vi "Graph Tool Testing1.vi"() -> ()   [LabVIEW 2019]
uses:
  Support/Graph Tools/Selection VIs/controls/CursorOptions.ctl
  <vilib>/Utility/miscctls.llb/LVRectTypeDef.ctl
  Support/Graph Tools/Selection VIs/controls/MarkerInfo.ctl
  Support/Graph Tools/Selection VIs/controls/markerType.ctl
  Support/Graph Tools/[Selection] Config.ctl
  <vilib>/Utility/miscctls.llb/LVPoint32TypeDef.ctl
  Support/Graph Tools/[Comment] Actions.ctl
  Support/Graph Tools/Selection Y-axis.vi
  Support/Graph Tools/Selection X-axis.vi
  Support/Graph Tools/Graph Tools.lvlib
panel:
  out "Display:Primary Workspace":T1
  out "Output Valid":bool
  out "X2":dbl
  out "X1":dbl
  in  "picture":picture
  in  "Cursor Options":T2={"font"={"Font Name"="Arial", "Size"=14, "Strikeout?"=FALSE, "Italic?"=FALSE, "Underline?"=FALSE, "Outline?"=FALSE, "Shadow?"=FALSE, "Bold?"=FALSE}, "size"=1, "Timestamp"=enum."at TOP", "Vertical Line?"=FALSE, "Horizontal Line?"=FALSE, "alignment(left, top)"={"horizontal"=enum."center", "vertical"=enum."center"}, "TextFormat"="%.3p %.3p %s", "time format (%H:%M:%S)"="%H:%M%:S"} {"size" min=1 max=50}
  out "Waveform Graph":T3(graph)
  out "XY Graph":cluster{i32[], dbl[]}[](graph)
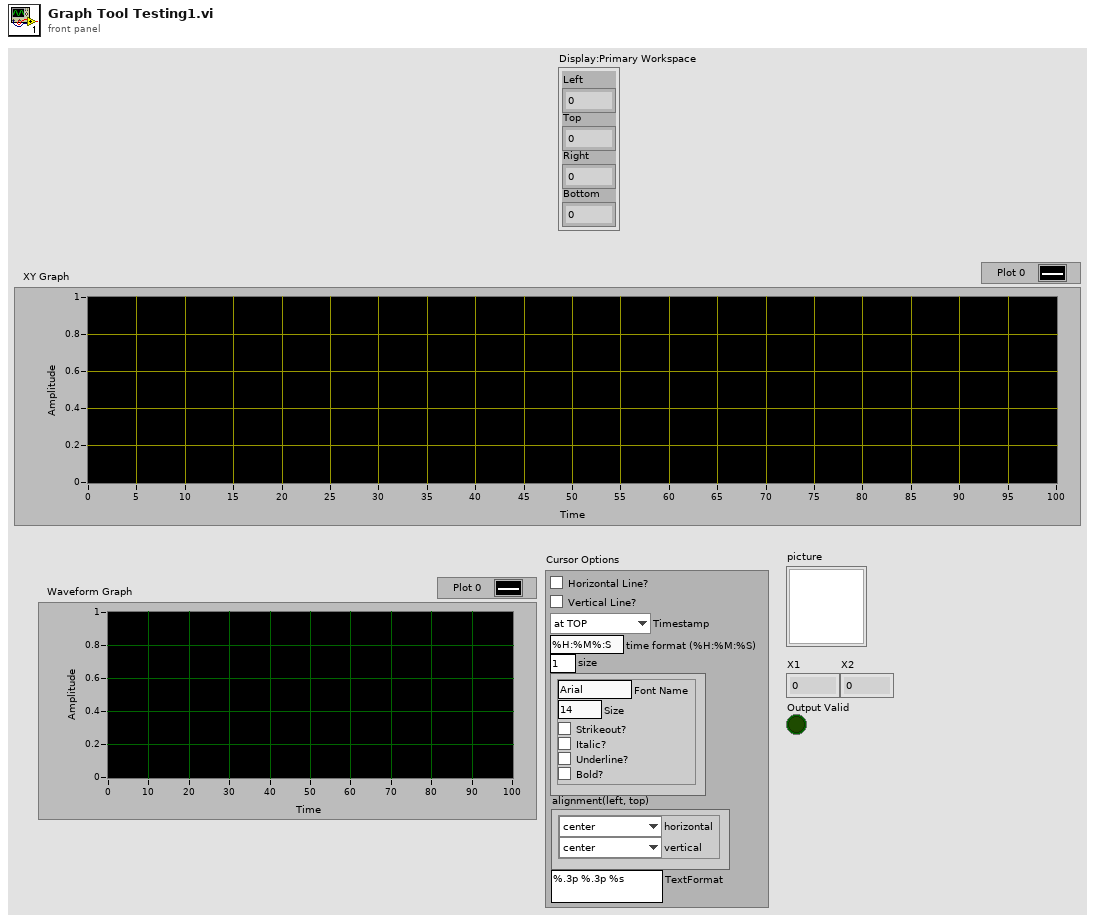
[diagram p1: front panel]
types:
  T1 = typedef "LVRectTypeDef.ctl" = cluster{"Left":i16, "Top":i16, "Right":i16, "Bottom":i16}
  T2 = typedef "CursorOptions.ctl" = cluster{"font":cluster{"Font Name":string, "Size":i16, "Strikeout?":bool, "Italic?":bool, "Underline?":bool, "Outline?":bool, "Shadow?":bool, "Bold?":bool}, "size":i16, "Timestamp":enum16{"at TOP", "at BOTTOM", "none"}, "Vertical Line?":bool, "Horizontal Line?":bool, "alignment(left, top)":cluster{"horizontal":enum16{"left", "center", "right"}, "vertical":enum16{"top", "center", "bottom"}}, "TextFormat":string, "time format (%H:%M:%S)":string}
  T3 = cluster{"number (0 to 1)":dbl, "number (0 to 1)":dbl, dbl[]}[]
  T4 = typedef "MarkerInfo.ctl" = cluster{"Type":T5, "X":dbl, "Y":dbl, "X2":dbl, "Y2":dbl, "Text":string}
  T5 = typedef "markerType.ctl" = enum16{"point", "arrow", "horiz", "vert", "vert range", "horiz range", "box"}
  T6 = cluster{"number (0 to 1)":dbl, "number (0 to 1)":dbl, dbl[]}
  T7 = typedef "Graph Tools.lvlib/[Comment] Actions.ctl" = enum16{"New Comment", "Refresh", "Clear", "Stop", "Test"}
  T8 = typedef "Graph Tools.lvlib/[Selection] Config.ctl" = cluster{"Selection":cluster{"caption":string, "Validaty Threshold":i32, "Color":u32, "Start Coords":T9}}
  T9 = typedef "LVPoint32TypeDef.ctl" = cluster{"Horizental":i32, "Vertical":i32}
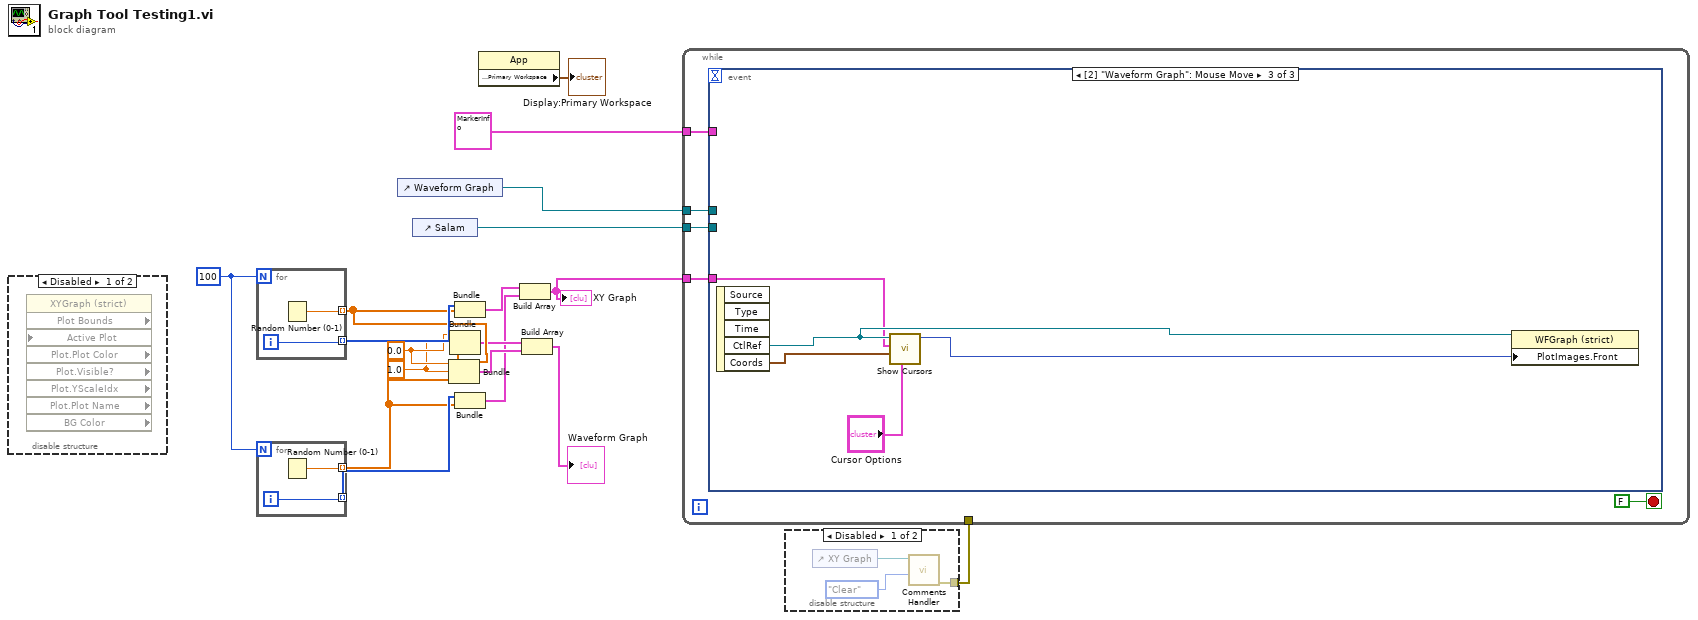
[diagram p0: block diagram]
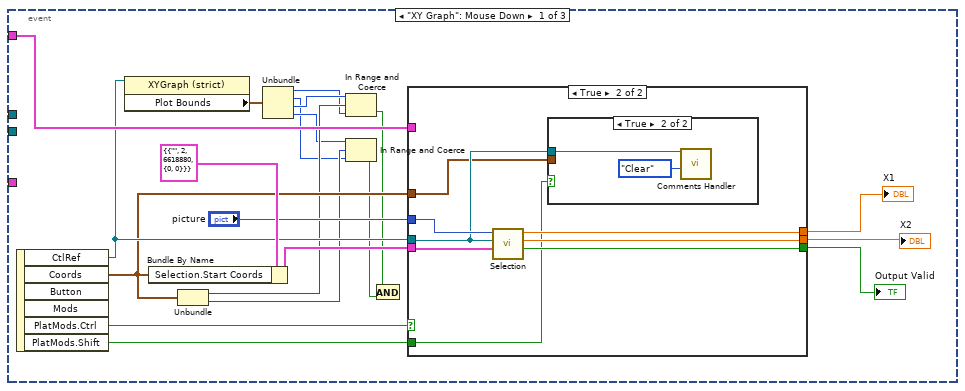
[diagram p4: hidden frame]
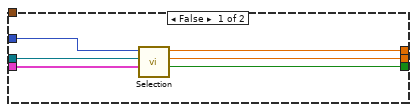
[diagram p5: hidden frame]
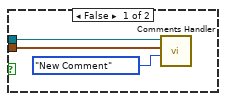
[diagram p6: hidden frame]
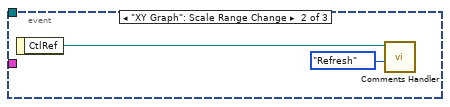
[diagram p7: hidden frame]
diagram:
  w10 = 1.0 ("number (0 to 1)")
  w11 = 0.0 ("number (0 to 1)")
  w16 = 100
  n1 = disable-structure shown="Disabled" {
    frame Disabled {
      n2 = property on="Property Node" class="XYGraph (strict)" props=["Plot Bounds", "Active Plot", "Plot", "Plot Color", "Plot", "Visible?", "Plot", "YScaleIdx", "Plot", "Plot Name", "BG Color"]() -> ()  [unwired: 3 in, 8 out]
    }
    frame Enabled {
    }
  }
  n3 = for {
    N: w16 -> [_]
    tunnel: [w20] -> w18 mode=indexing
    tunnel: [w19] -> w9 mode=indexing
    i -> [w20]
    n4 = Random Number (0-1)() -> (number: 0 to 1=w19:dbl)
  }
  n5 = for {
    N: w16 -> [_]
    tunnel: [w22] -> w17 mode=indexing
    tunnel: [w21] -> w13 mode=indexing
    i -> [w22]
    n6 = Random Number (0-1)() -> (number: 0 to 1=w21:dbl)
  }
  n7 = control-ref of="Waveform Graph"() -> (w6:refnum<vi>)
  n8 = control-ref of="Salam"() -> (w14:refnum<vi>)
  n9 = Bundle("number (0 to 1)"=w11, "number (0 to 1)"=w10, w13) -> (w12:T6)  [unwired: 1 in]
  n10 = Bundle("number (0 to 1)"=w11, "number (0 to 1)"=w10, w9) -> (w8:T6)  [unwired: 1 in]
  n11 = Bundle(w18, w9) -> (w15:cluster{i32[], dbl[]})  [unwired: 1 in]
  n12 = Bundle(w17, w13) -> (w7:cluster{i32[], dbl[]})  [unwired: 1 in]
  n13 = property class="App"() -> ("Display:Primary Workspace"=→"Display:Primary Workspace":T1)  [unwired: 2 in, 2 out]
  n14 = Build Array(w15, w7) -> (w4:cluster{i32[], dbl[]}[])
  "XY Graph" <- w4
  n15 = Build Array(w8, w12) -> (→"Waveform Graph":T3)
  n16 = disable-structure shown="Disabled" {
    disable-tunnel: [w23 _] -> w1
    frame Disabled {
      n17 = control-ref of="XY Graph"() -> (w25:refnum<vi>)
      n18 = call "Comments Handler.vi"("Action"=[Comment]_Actions."Clear", "GrphChrt"=w25) -> ("error out"=w23:errorcluster)  [unwired: 9 in]
    }
    frame Enabled {
    }
  }
  n19 = while {
    tunnel: w14 -> [w29]
    tunnel: w6 -> [w28]
    tunnel: w4 -> [w27]
    tunnel: T4 {"Type"=enum."vert", "X"=2.0, "Y"=2.0, "X2"=2.0, "Y2"=2.0, "Text"="Drag and click to\nposition a marker"} ("Marker") -> [w26]
    tunnel: w1 -> [_]
    stop <- FALSE stop-if-true
    n20 = event shown="[2] \"Waveform Graph\": Mouse Move" {
      selector: _ -> [_ _ _]
      dyn-events: _ -> [_ _ _]
      timeout: _ -> [_ _ _]
      tunnel: w29 -> [_ _ _]
      tunnel: w28 -> [_ _ _]
      tunnel: w27 -> [_ _ w72]
      tunnel: w26 -> [w44 _ _]
      event "XY Graph": Mouse Down {
        n21 = event-data() -> ("CtlRef"=w42:refnum<vi>, "Coords"=w40:T9, "PlatMods.Ctrl"=w31:bool, "PlatMods.Shift"=w43:bool)  [unwired: 1 in, 2 out]
        n22 = property class="XYGraph (strict)"(reference=w42) -> ("Plot Bounds"=w41:T1)  [unwired: 1 in, 2 out]
        n23 = Bundle By Name(cluster=T8 {"Selection"={"caption"="", "Validaty Threshold"=2, "Color"=6618880, "Start Coords"={"Horizental"=0, "Vertical"=0}}} ("Config"), "Selection.Start Coords"=w40) -> (w49:T8)
        n24 = Unbundle(w40) -> ("Horizontal"=w39:i32, "Vertical"=w36:i32)
        n25 = Unbundle(w41) -> ("Left"=w37:i16, "Top"=w34:i16, "Right"=w38:i16, "Bottom"=w35:i16)
        n26 = In Range and Coerce(upper limit=w38, x=w39, lower limit=w37) -> (In Range?=w33:bool)  [unwired: 1 out]
        n27 = In Range and Coerce(upper limit=w35, x=w36, lower limit=w34) -> (In Range?=w32:bool)  [unwired: 1 out]
        n28 = And(x=w33, y=w32) -> ()  [unwired: 1 out]
        n29 = case shown="True" w31 {
          tunnel: w49 -> [w56 w64]
          tunnel: w42 -> [w55 w59]
          tunnel: "picture" -> [w54 w60]
          tunnel: [w53 w62] -> w47
          tunnel: [w52 w61] -> w46
          tunnel: [w51 w63] -> w45
          tunnel: w44 -> [_ _]
          tunnel: w40 -> [_ w58]
          tunnel: w43 -> [_ w57]
          frame False {
            n30 = call-poly "Selection.vi"("Config"=w56, "GrphChrt Refnum"=w55, "picture"=w54) -> ("Output Valid"=w51:bool, "Y2"=w52:dbl, "Y1"=w53:dbl)  [unwired: 5 in, 1 out]
          }
          frame True {
            n31 = call-poly "Selection.vi"("Config"=w64, "GrphChrt Refnum"=w59, "picture"=w60) -> ("Output Valid"=w63:bool, "X2"=w61:dbl, "X1"=w62:dbl)  [unwired: 5 in, 1 out]
            n32 = case shown="True" w57 {
              tunnel: w59 -> [w67 w69]
              tunnel: w58 -> [w66 _]
              frame False {
                n33 = call "Comments Handler.vi"("Action"=[Comment]_Actions."New Comment", "Coords"=w66, "GrphChrt"=w67) -> ()  [unwired: 8 in, 1 out]
              }
              frame True {
                n34 = call "Comments Handler.vi"("Action"=[Comment]_Actions."Clear", "GrphChrt"=w69) -> ()  [unwired: 9 in, 1 out]
              }
            }
          }
        }
        "X1" <- w47
        "X2" <- w46
        "Output Valid" <- w45
      }
      event "XY Graph": Scale Range Change {
        n35 = event-data() -> ("CtlRef"=w71:refnum<vi>)  [unwired: 1 in]
        n36 = call "Comments Handler.vi"("Action"=[Comment]_Actions."Refresh", "GrphChrt"=w71) -> ()  [unwired: 9 in, 1 out]
      }
      event "Waveform Graph": Mouse Move {
        n37 = event-data() -> ("CtlRef"=w73:refnum<vi>, "Coords"=w76:T9)  [unwired: 1 in, 3 out]
        n38 = call "Show Cursors.vi"("Cursor Options"="Cursor Options", "Coords"=w76, "Graph Data"=w72, "Grapg"=w73) -> ("output picture"=w74:picture)  [unwired: 6 in, 1 out]
        n39 = property class="WFGraph (strict)"(reference=w73, "PlotImages.Front"=w74) -> ()  [unwired: 1 in, 2 out]
      }
    }
  }
